vi "Destroy Sync Tool.vi"(8 "error in (no error)":errorcluster, 11 "CD Build Tools in":refnum<class "Project Sync Tools.lvclass">) -> (0 "error out":errorcluster)   [LabVIEW 2019, in "Project Sync Tools.lvclass"]
uses:
  Project Sync Tools.lvclass
  Project Sync Tools.lvclass/Project Sync Tools.ctl
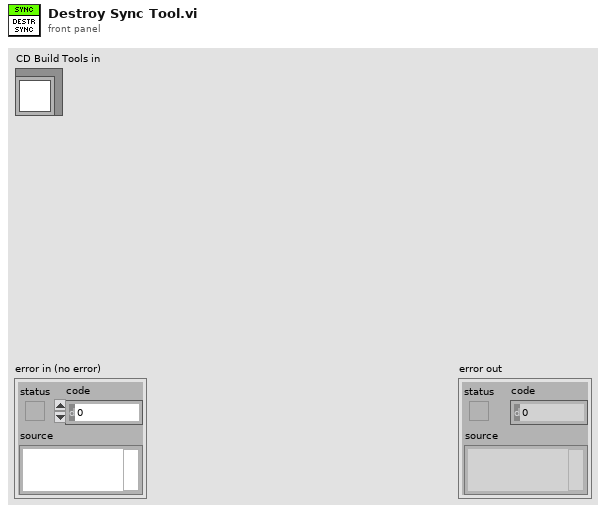
[diagram p1: front panel]
types:
  T1 = typedef "Project Sync Tools.lvclass/BuildSpec Parameters.ctl" = cluster{"BuildSpec Ref":refnum<vi>, "Target Name":string, "Build Spec Name":string, "Tags":string[], "Tag Values":variant[]}
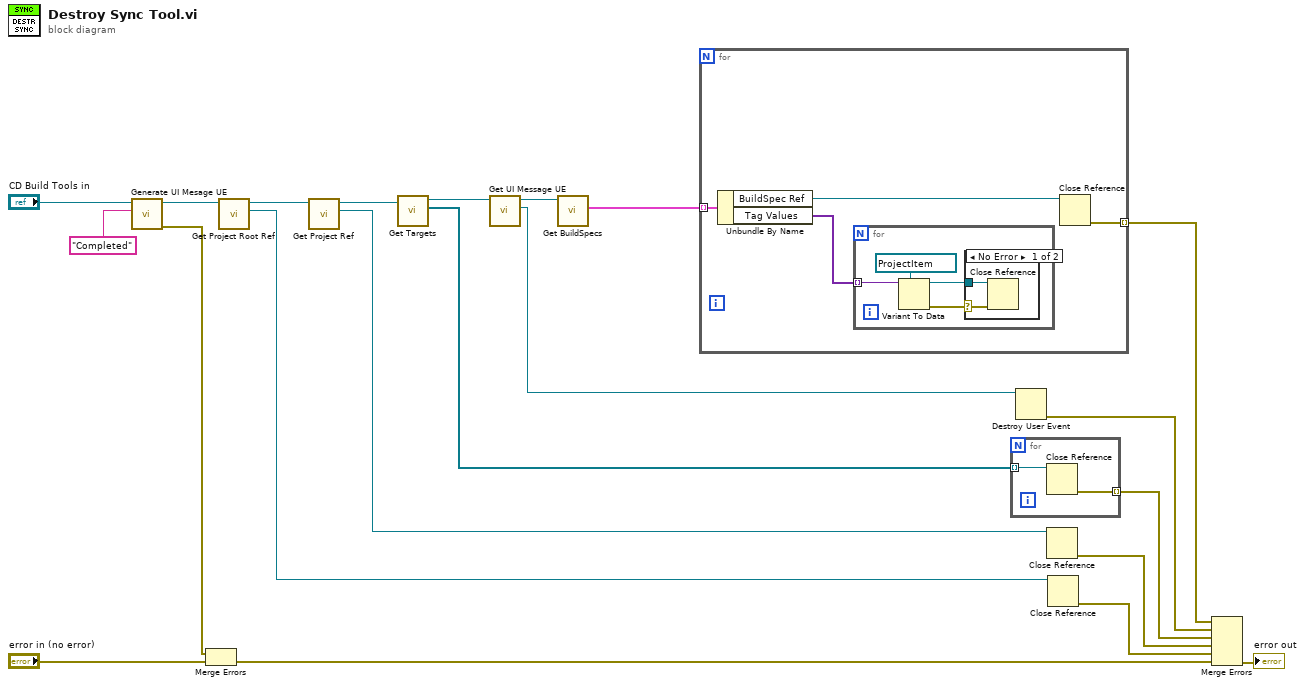
[diagram p0: block diagram]
diagram:
  n1 = call "Generate UI Mesage UE.vi"("UI Message"="Completed", "Project Sync Tools in"="CD Build Tools in") -> ("error out"=w1:errorcluster, "Project Sync Tools out"=w5:refnum<class "Project Sync Tools.lvclass">)  [unwired: 8 in]
  n2 = Merge Errors(w1, "error in (no error)") -> (w2:errorcluster)
  n3 = call "Get Project Root Ref.vi"("CD Build Tools in"=w5) -> ("Project Root Ref"=w20:refnum<vi>, "CD Build Tools out"=w21:refnum<class "Project Sync Tools.lvclass">)  [unwired: 9 in]
  n4 = call "Get Project Ref.vi"("CD Build Tools in"=w21) -> ("Project Ref"=w19:refnum<vi>, "CD Build Tools out"=w15:refnum<class "Project Sync Tools.lvclass">)  [unwired: 9 in]
  n5 = call "Get Targets.vi"("Project Sync Tools in"=w15) -> ("Targets"=w14:refnum<vi>[], "Project Sync Tools out"=w11:refnum<class "Project Sync Tools.lvclass">)  [unwired: 9 in]
  n6 = call "Get UI Message UE.vi"("Project Sync Tools in"=w11) -> ("UI Message UE"=w9:refnum<user-event>, "Project Sync Tools out"=w10:refnum<class "Project Sync Tools.lvclass">)  [unwired: 9 in]
  n7 = call "Get BuildSpecs.vi"("Project Sync Tools in"=w10) -> ("BuildSpecs"=w12:T1[])  [unwired: 9 in, 1 out]
  n8 = for {
    tunnel: w12 -> [w25] mode=indexing
    tunnel: [w24] -> w7 mode=indexing
    n9 = Unbundle By Name(w25) -> ("BuildSpec Ref"=w23:refnum<vi>, "Tag Values"=w22:variant[])
    n10 = for {
      tunnel: w22 -> [w28] mode=indexing
      n11 = Variant To Data(type=refnum<vi> refnum ("BuildSpec Ref"), Variant=w28) -> (data=w26:refnum<vi>, error out=w27:errorcluster)  [unwired: 1 in]
      n12 = case shown="No Error" w27 {
        selector: w27 -> [w31 _]
        tunnel: w26 -> [w30 _]
        frame No Error {
          n13 = Close Reference(reference=w30, error in (no error)=w31) -> ()  [unwired: 1 out]
        }
        frame Error {
        }
      }
    }
    n14 = Close Reference(reference=w23) -> (error out=w24:errorcluster)  [unwired: 1 in]
  }
  n15 = for {
    tunnel: w14 -> [w33] mode=indexing
    tunnel: [w32] -> w13 mode=indexing
    n16 = Close Reference(reference=w33) -> (error out=w32:errorcluster)  [unwired: 1 in]
  }
  n17 = Destroy User Event(user event=w9) -> (error out=w8:errorcluster)  [unwired: 1 in]
  n18 = Close Reference(reference=w19) -> (error out=w17:errorcluster)  [unwired: 1 in]
  n19 = Close Reference(reference=w20) -> (error out=w18:errorcluster)  [unwired: 1 in]
  n20 = Merge Errors(w7, w8, w13, w17, w18, w2) -> (→"error out":errorcluster)
